vi "_Clear Numeric - FP.vi"(0 "GObject in":refnum<vi>, 5 "error in (no error)":errorcluster) -> (14 "changed?":bool, 19 "error out":errorcluster)   [LabVIEW 2017, in "QD_Erease Data.lvlib"]
uses:
  QD_Erease Data.lvlib
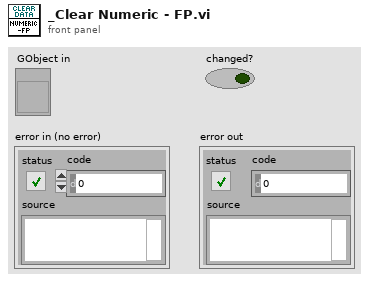
[diagram p1: front panel]
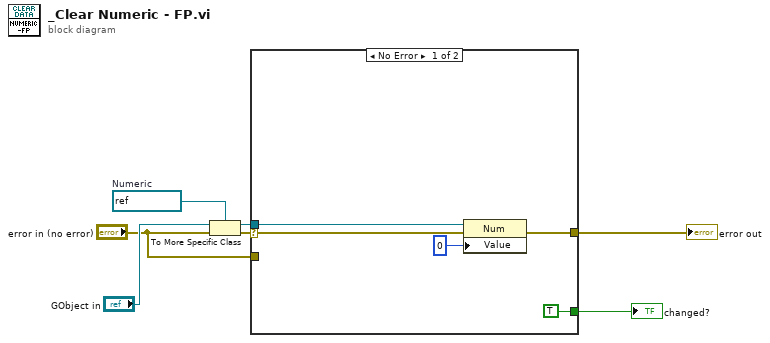
[diagram p0: block diagram]
diagram:
  w1 = refnum<vi> refnum  # Numeric
  n1 = To More Specific Class(target class=w1, reference="GObject in", error in="error in (no error)") -> (specific class reference=w3:refnum<vi>, error out=w4:errorcluster)
  n2 = case shown="No Error" w4 {
    selector: w4 -> [w9 _]
    tunnel: [w12 w13] -> w2
    tunnel: w3 -> [w10 _]
    tunnel: "error in (no error)" -> [_ w13]
    tunnel: [TRUE _] -> w7
    frame No Error {
      n3 = property class="Num"(reference=w10, error in=w9, "Value"=0) -> (error out=w12:errorcluster)  [unwired: 1 out]
    }
    frame Error {
    }
  }
  "changed?" <- w7
  "error out" <- w2
